vi "Launcher.vi"   [LabVIEW 2016, in "WS Full LabVIEW Test.lvlib"]
uses:
  WS Full LabVIEW Test.lvlib
  <vilib>/ActorFramework/Actor/Actor.lvclass
  WebSocket Server/WebSocket Server.lvclass
  WebSocket Server Messages/Add Service Msg/Add Service Msg.lvclass
  WS Test Server/WS Test Server.lvclass
  WS Test Server Messages/Server Connection Handler Msg/Server Connection Handler Msg.lvclass
  WS Test Client/WS Test Client.lvclass
  WebSocket Server/typedefs/Listener Settings.ctl
  C:/Program Files (x86)/National Instruments/LabVIEW 2016/vi.lib/ActorFramework/Actor/Actor.lvclass
  C:/Projects/Shared Libraries/WebSocket Actor/WebSocket Actor/Abstract Messages/WebSocket Connection Handler Msg/WebSocket Connection Handler Msg.lvclass
  C:/Program Files (x86)/National Instruments/LabVIEW 2016/vi.lib/ActorFramework/Message/Message.lvclass
types:
  T1 = typedef "WebSocket Actors.lvlib/WebSocket Server.lvclass/Listener Settings.ctl" = cluster{"resolve remote address (T)":bool, "timeout ms (-1)":i32, "net address":u32, "port":u16}
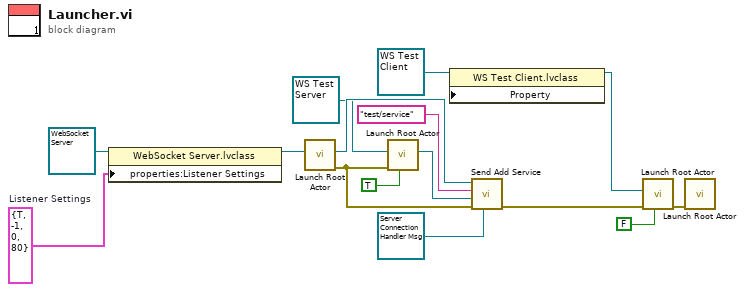
[diagram p0: block diagram]
diagram:
  w2 = T1 {"resolve remote address (T)"=TRUE, "timeout ms (-1)"=-1, "net address"=0, "port"=80}  # Listener Settings
  n1 = property class="WebSocket Server.lvclass"(reference=refnum<class "WebSocket Server.lvclass"> refnum ("WebSocket Actors.lvlib:WebSocket Server.lvclass"), "properties:Listener Settings"=w2) -> (reference out=w3:refnum<class "WebSocket Server.lvclass">)  [unwired: 1 in, 1 out]
  n2 = call <vilib>:"Launch Root Actor.vi"("Actor"=w3) -> ("error out"=w10:errorcluster, "Actor's Enqueuer"=w12:refnum<class "Message Enqueuer.lvclass">)  [unwired: 9 in]
  n3 = call <vilib>:"Launch Root Actor.vi"("Open Actor Core front panel? (F)"=TRUE, "error in (no error)"=w10, "Actor"=refnum<class "WS Test Server.lvclass"> refnum ("WS Full LabVIEW Test.lvlib:WS Test Server.lvclass")) -> ("Actor's Enqueuer"=w9:refnum<class "Message Enqueuer.lvclass">)  [unwired: 7 in, 1 out]
  n4 = property class="WS Test Client.lvclass" props=[](reference=refnum<class "WS Test Client.lvclass"> refnum ("WS Full LabVIEW Test.lvlib:WS Test Client.lvclass")) -> (reference out=w1:refnum<class "WS Test Client.lvclass">)  [unwired: 2 in, 1 out]
  n5 = call "Send Add Service.vi"("WebSocket Data Handler"=refnum<class "Server Connection Handler Msg.lvclass"> refnum ("WS Full LabVIEW Test.lvlib:Server Connection Handler Msg.lvclass"), "error in (no error)"=w10, "Subscriber Enqueuer"=w9, "Service Name"="test/service", "Message Enqueuer in"=w12) -> ("error out"=w5:errorcluster)  [unwired: 5 in, 1 out]
  n6 = call <vilib>:"Launch Root Actor.vi"("Open Actor Core front panel? (F)"=FALSE, "error in (no error)"=w5, "Actor"=w1) -> ("error out"=w15:errorcluster)  [unwired: 7 in, 1 out]
  n7 = call <vilib>:"Launch Root Actor.vi"("error in (no error)"=w15) -> ()  [unwired: 9 in, 2 out]
